vi "Laser 1 Update status selected L3.vi"(7 "Array":bool[](array[boolean]), 9 "Numeric in":dbl[](array[numeric]), 10 "Ls1 User Controls":T1, 11 "I/p string(s)":string[](array[string])) -> (2 "Numeric out":dbl, 3 "Array":errorcluster[](array[cluster]))   [LabVIEW 2017]
uses:
  Type Defs/Ls1 User Controls.ctl
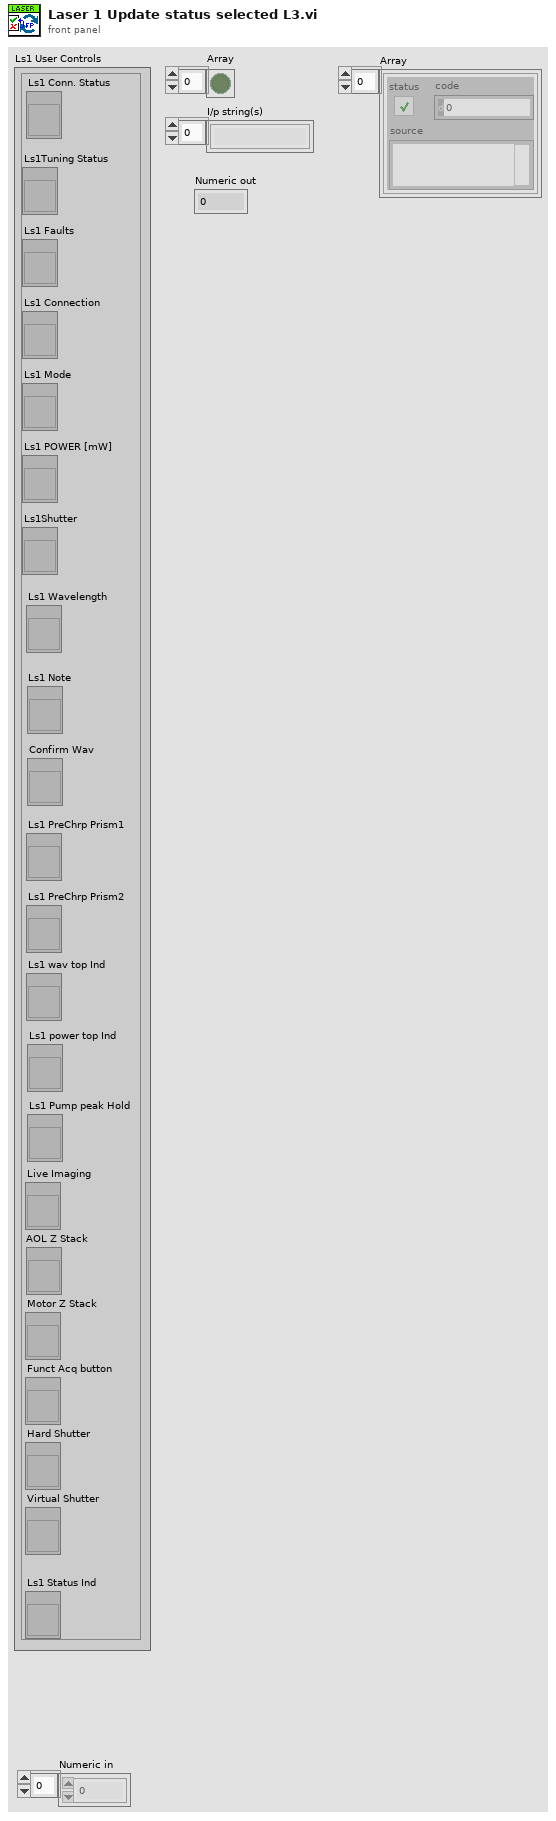
[diagram p1: front panel]
types:
  T1 = typedef "Ls1 User Controls.ctl" = cluster{"Ls1 Conn. Status":refnum<vi>, "Ls1Tuning Status":refnum<vi>, "Ls1 Faults":refnum<vi>, "Ls1 Connection":refnum<vi>, "Ls1 Mode":refnum<vi>, "Ls1 POWER [mW]":refnum<vi>, "Ls1Shutter":refnum<vi>, "Ls1 Wavelength":refnum<vi>, "Ls1 Note":refnum<vi>, "Confirm Wav":refnum<vi>, "Ls1 PreChrp Prism1":refnum<vi>, "Ls1 PreChrp Prism2":refnum<vi>, "Ls1 wav top Ind":refnum<vi>, "Ls1 power top Ind":refnum<vi>, "Ls1 Pump peak Hold":refnum<vi>, "Live Imaging":refnum<vi>, "AOL Z Stack":refnum<vi>, "Motor Z Stack":refnum<vi>, "Funct Acq button":refnum<vi>, "Hard Shutter":refnum<vi>, "Virtual Shutter":refnum<vi>, "Ls1 Status Ind":refnum<vi>}
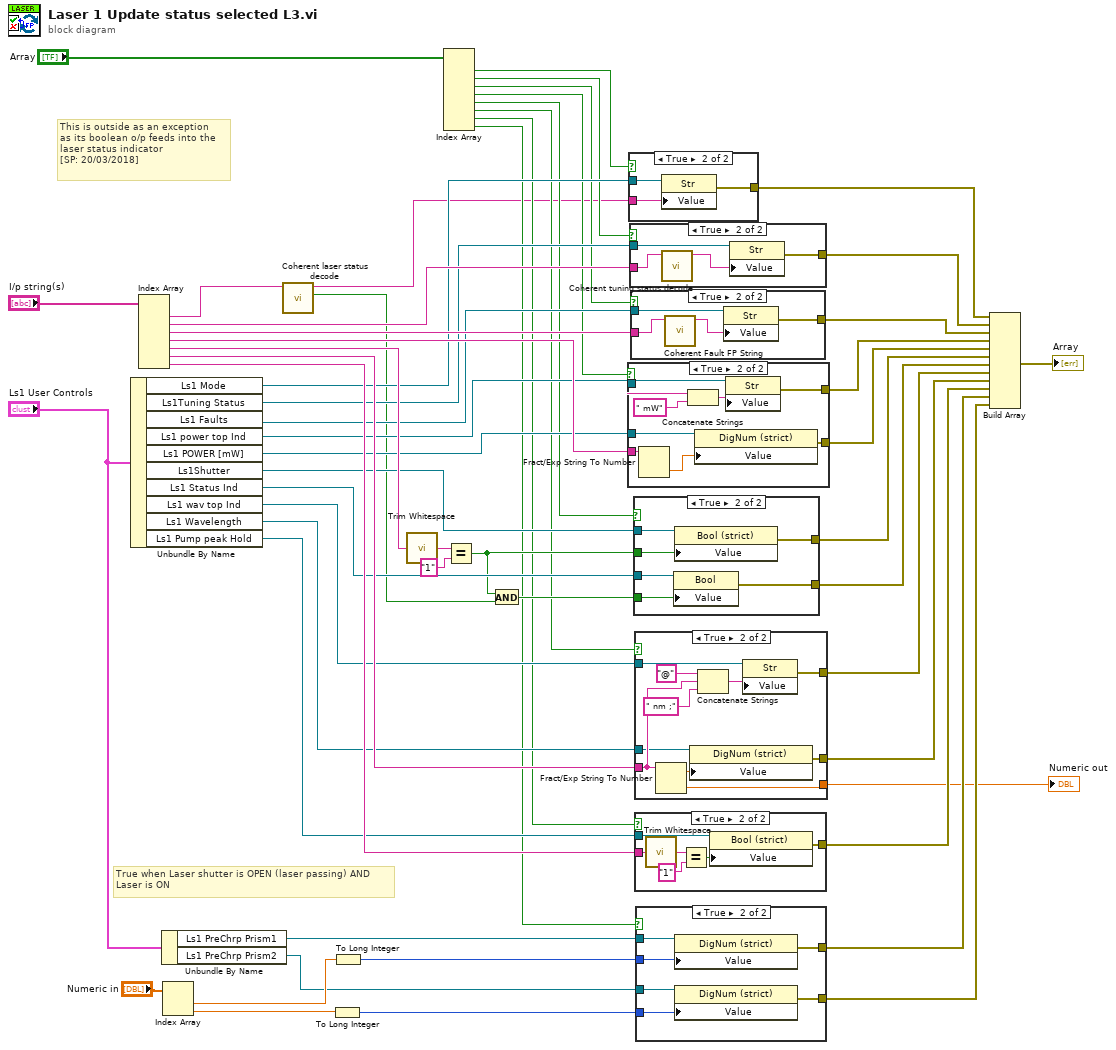
[diagram p0: block diagram]
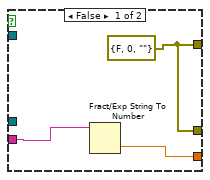
[diagram p2: hidden frame]
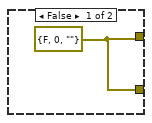
[diagram p3: hidden frame]
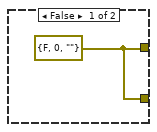
[diagram p4: hidden frame]
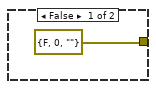
[diagram p5: hidden frame]
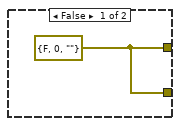
[diagram p6: hidden frame]
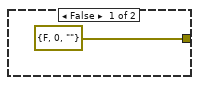
[diagram p7: hidden frame]
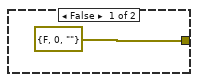
[diagram p8: hidden frame]
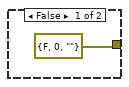
[diagram p9: hidden frame]
diagram:
  # "This is outside as an exception\nas its boolean o/p feeds into the\nlaser status indicator\n[SP: 20/03/2018]"
  # "True when Laser shutter is OPEN (laser passing) AND\nLaser is ON"
  n1 = Unbundle By Name("Ls1 User Controls") -> ("Ls1 Mode"=w14:refnum<vi>, "Ls1Tuning Status"=w15:refnum<vi>, "Ls1 Faults"=w16:refnum<vi>, "Ls1 power top Ind"=w20:refnum<vi>, "Ls1 POWER [mW]"=w21:refnum<vi>, "Ls1Shutter"=w23:refnum<vi>, "Ls1 Status Ind"=w29:refnum<vi>, "Ls1 wav top Ind"=w30:refnum<vi>, "Ls1 Wavelength"=w31:refnum<vi>, "Ls1 Pump peak Hold"=w33:refnum<vi>)
  n2 = Index Array(array="I/p string(s)") -> (element #1=w3:string, element #2=w18:string, element #3=w19:string, element #4=w22:string, element #5=w24:string, element #6=w32:string, element #7=w34:string)  [unwired: 7 in]
  n3 = Unbundle By Name("Ls1 User Controls") -> ("Ls1 PreChrp Prism1"=w36:refnum<vi>, "Ls1 PreChrp Prism2"=w37:refnum<vi>)
  n4 = Index Array(array="Numeric in") -> (element #1=w40:dbl, element #2=w42:dbl)  [unwired: 2 in]
  n5 = call "Coherent laser status decode.vi"("I/p String"=w3) -> ("Boolean"=w1:bool, "String"=w2:string)  [unwired: 9 in]
  n6 = To Long Integer(number=w42) -> (32bit integer=w41:i32)
  n7 = To Long Integer(number=w40) -> (32bit integer=w39:i32)
  n8 = call <vilib>:"Trim Whitespace.vi"("string"=w24) -> ("trimmed string"=w25:string)  [unwired: 1 in]
  n9 = Index Array(array="Array") -> (element #1=w12:bool, element #2=w10:bool, element #3=w9:bool, element #4=w8:bool, element #5=w7:bool, element #6=w6:bool, element #7=w5:bool, element #8=w4:bool)  [unwired: 8 in]
  n10 = Equal?(x=w25, y="1") -> (x = y?=w28:bool)
  n11 = And(x=w28, y=w1) -> (x .and. y?=w27:bool)
  n12 = case shown="True" w8 {
    tunnel: [w56 w64] -> w47
    tunnel: [w56 w63] -> w46
    tunnel: w22 -> [_ w62]
    tunnel: w21 -> [_ w61]
    tunnel: w20 -> [_ w60]
    frame False {
      w56 = errorcluster {"status"=FALSE, "code"=0, "source"=""} ("error out")
    }
    frame True {
      n13 = Fract/Exp String To Number(string=w62) -> (number=w59:dbl)  [unwired: 3 in, 1 out]
      n14 = Concatenate Strings(w62, " mW" ("string")) -> (w58:string)
      n15 = property class="DigNum (strict)"(reference=w61, "Value"=w59) -> (error out=w64:errorcluster)  [unwired: 1 in, 1 out]
      n16 = property class="Str"(reference=w60, "Value"=w58) -> (error out=w63:errorcluster)  [unwired: 1 in, 1 out]
    }
  }
  n17 = case shown="True" w12 {
    tunnel: [errorcluster {"status"=FALSE, "code"=0, "source"=""} ("error out") w68] -> w43
    tunnel: w2 -> [_ w67]
    tunnel: w14 -> [_ w66]
    frame False {
    }
    frame True {
      n18 = property class="Str"(reference=w66, "Value"=w67) -> (error out=w68:errorcluster)  [unwired: 1 in, 1 out]
    }
  }
  n19 = case shown="True" w10 {
    tunnel: [errorcluster {"status"=FALSE, "code"=0, "source"=""} ("error out") w73] -> w44
    tunnel: w18 -> [_ w71]
    tunnel: w15 -> [_ w72]
    frame False {
    }
    frame True {
      n20 = call "Coherent tuning status decode.vi"("I/p String"=w71) -> ("O/P String"=w70:string)  [unwired: 10 in]
      n21 = property class="Str"(reference=w72, "Value"=w70) -> (error out=w73:errorcluster)  [unwired: 1 in, 1 out]
    }
  }
  n22 = case shown="True" w9 {
    tunnel: [errorcluster {"status"=FALSE, "code"=0, "source"=""} ("error out") w78] -> w45
    tunnel: w19 -> [_ w76]
    tunnel: w16 -> [_ w77]
    frame False {
    }
    frame True {
      n23 = call "Coherent Fault FP String.vi"("I/p String"=w76) -> ("O/P String"=w75:string)  [unwired: 10 in]
      n24 = property class="Str"(reference=w77, "Value"=w75) -> (error out=w78:errorcluster)  [unwired: 1 in, 1 out]
    }
  }
  n25 = case shown="True" w7 {
    tunnel: [w79 w85] -> w49
    tunnel: [w79 w84] -> w48
    tunnel: w29 -> [_ w83]
    tunnel: w28 -> [_ w82]
    tunnel: w27 -> [_ w81]
    tunnel: w23 -> [_ w80]
    frame False {
      w79 = errorcluster {"status"=FALSE, "code"=0, "source"=""} ("error out")
    }
    frame True {
      n26 = property class="Bool"(reference=w83, "Value"=w81) -> (error out=w85:errorcluster)  [unwired: 1 in, 1 out]
      n27 = property class="Bool (strict)"(reference=w80, "Value"=w82) -> (error out=w84:errorcluster)  [unwired: 1 in, 1 out]
    }
  }
  n28 = case shown="True" w6 {
    tunnel: [w88 w97] -> w51
    tunnel: [w88 w96] -> w50
    tunnel: [w86 w95] -> w35
    tunnel: w32 -> [w87 w94]
    tunnel: w31 -> [_ w93]
    tunnel: w30 -> [_ w92]
    frame False {
      w88 = errorcluster {"status"=FALSE, "code"=0, "source"=""} ("error out")
      n29 = Fract/Exp String To Number(string=w87) -> (number=w86:dbl)  [unwired: 3 in, 1 out]
    }
    frame True {
      n30 = Fract/Exp String To Number(string=w94) -> (number=w95:dbl)  [unwired: 3 in, 1 out]
      n31 = property class="DigNum (strict)"(reference=w93, "Value"=w95) -> (error out=w97:errorcluster)  [unwired: 1 in, 1 out]
      n32 = Concatenate Strings("@" ("string"), w94, " nm ;" ("string")) -> (w90:string)
      n33 = property class="Str"(reference=w92, "Value"=w90) -> (error out=w96:errorcluster)  [unwired: 1 in, 1 out]
    }
  }
  "Numeric out" <- w35
  n34 = case shown="True" w5 {
    tunnel: [errorcluster {"status"=FALSE, "code"=0, "source"=""} ("error out") w104] -> w52
    tunnel: w34 -> [_ w103]
    tunnel: w33 -> [_ w101]
    frame False {
    }
    frame True {
      n35 = call <vilib>:"Trim Whitespace.vi"("string"=w103) -> ("trimmed string"=w99:string)  [unwired: 1 in]
      n36 = Equal?(x=w99, y="1") -> (x = y?=w102:bool)
      n37 = property class="Bool (strict)"(reference=w101, "Value"=w102) -> (error out=w104:errorcluster)  [unwired: 1 in, 1 out]
    }
  }
  n38 = case shown="True" w4 {
    tunnel: [w105 w111] -> w55
    tunnel: [w105 w110] -> w54
    tunnel: w41 -> [_ w109]
    tunnel: w39 -> [_ w108]
    tunnel: w37 -> [_ w107]
    tunnel: w36 -> [_ w106]
    frame False {
      w105 = errorcluster {"status"=FALSE, "code"=0, "source"=""} ("error out")
    }
    frame True {
      n39 = property class="DigNum (strict)"(reference=w106, "Value"=w108) -> (error out=w110:errorcluster)  [unwired: 1 in, 1 out]
      n40 = property class="DigNum (strict)"(reference=w107, "Value"=w109) -> (error out=w111:errorcluster)  [unwired: 1 in, 1 out]
    }
  }
  n41 = Build Array(w43, w44, w45, w46, w47, w48, w49, w50, w51, w52, w54, w55) -> (→"Array":errorcluster[])
